vi "Normalize Forecast and Price Data.vi"(9 "PV Forecast Waveforms Array":waveform(dbl)[](array[waveform]), 10 "Price Forecast Waveform":waveform(dbl), 11 "Load Forecast Waveforms Array":waveform(dbl)[](array[waveform])) -> (0 "Load Magnitudes":dbl[][](array[numeric]), 1 "PV Magnitudes":dbl[][](array[numeric]), 2 "Price Magnitudes":dbl[][](array[numeric]), 3 "Normalized dt":dbl)   [LabVIEW 2018, in "Generic Optimization Actor.lvlib" / "Generic Optimization.lvclass"]
doc: "Normalizes all forecast waveforms to have the same t0 and dt. Also trims all waveforms to be the same length."
uses:
  Generic Optimization.lvclass
  Utilities/Forecast-Waveform-Equalizer/Waveform Equalizer/subVIs/Get Target dt.vi
  Utilities/Forecast-Waveform-Equalizer/Waveform Equalizer/subVIs/Time Slide and Interpolate.vi
  Utilities/Forecast-Waveform-Equalizer/Waveform Equalizer/subVIs/Get Target t0.vi
  Utilities/Forecast-Waveform-Equalizer/Waveform Equalizer/subVIs/Get Minimum Length.vi
  Utilities/Forecast-Waveform-Equalizer/Waveform Equalizer/subVIs/Interpolate.vi
  Utilities/Forecast-Waveform-Equalizer/Waveform Equalizer/subVIs/Greater or Equal with Epsilon.vi
  Utilities/Forecast-Waveform-Equalizer/Waveform Equalizer/Waveform Equalizer.lvlib
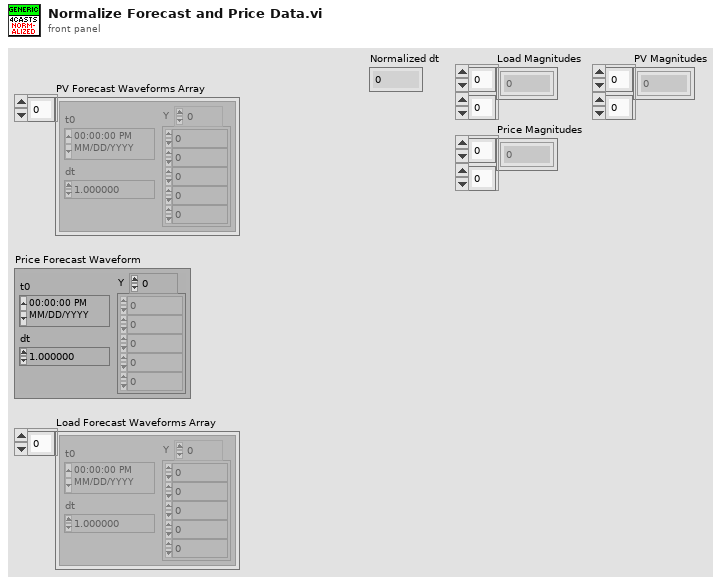
[diagram p1: front panel]
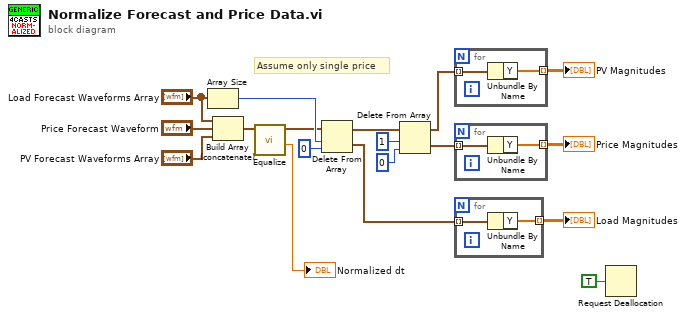
[diagram p0: block diagram]
diagram:
  # "Assume only single price"
  n1 = Array Size(array="Load Forecast Waveforms Array") -> (size(s)=w14:i32)
  n2 = Build Array (concatenate)("Load Forecast Waveforms Array", "Price Forecast Waveform", "PV Forecast Waveforms Array") -> (w11:waveform(dbl)[])
  n3 = call "Equalize.vi"("Analog Waveform Array in"=w11) -> ("Target dt"=→"Normalized dt":dbl, "Analog Waveform Array out"=w13:waveform(dbl)[])  [unwired: 9 in]
  n4 = Delete From Array(array=w13, length=w14, index=0) -> (deleted portion=w8:waveform(dbl)[], array with subset deleted=w16:waveform(dbl)[])
  n5 = Delete From Array(array=w16, length=1, index=0) -> (deleted portion=w6:waveform(dbl)[], array with subset deleted=w4:waveform(dbl)[])
  n6 = for {
    tunnel: w4 -> [w20] mode=indexing
    tunnel: [w19] -> w3 mode=indexing
    n7 = Unbundle By Name(w20) -> ("Y"=w19:dbl[])
  }
  "PV Magnitudes" <- w3
  n8 = for {
    tunnel: w6 -> [w22] mode=indexing
    tunnel: [w21] -> w5 mode=indexing
    n9 = Unbundle By Name(w22) -> ("Y"=w21:dbl[])
  }
  "Price Magnitudes" <- w5
  n10 = for {
    tunnel: w8 -> [w24] mode=indexing
    tunnel: [w23] -> w7 mode=indexing
    n11 = Unbundle By Name(w24) -> ("Y"=w23:dbl[])
  }
  "Load Magnitudes" <- w7
  n12 = Request Deallocation(TRUE ("flag")) -> ()
